vi "Is Error.vi"(8 "error in":errorcluster, 11 "Queue in":refnum<queue>) -> (0 "error out":errorcluster, 3 "Queue out":refnum<queue>)   [LabVIEW 2018, in "Module A.lvlib"]
doc: "Sends state machine to error case."
uses:
  Module A.lvlib
  ctl/Message Data--cluster.ctl
  ctl/State--enum.ctl
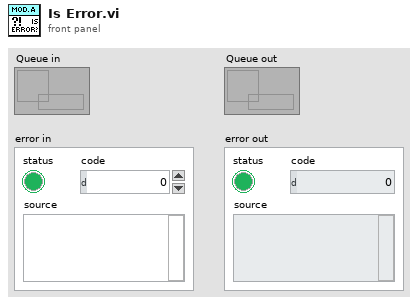
[diagram p1: front panel]
types:
  T1 = typedef "Module A.lvlib/State--enum.ctl" = enum16{"Initialize", "Error", "Shut Down", "Stop Module", "---", "Template", "Shut Module B", "Start Module B"}
  T2 = typedef "Module A.lvlib/Message Data--cluster.ctl" = cluster{"State":T1, "Data":variant}
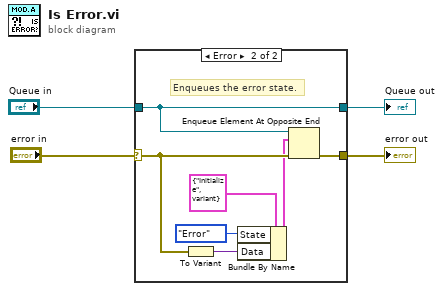
[diagram p0: block diagram]
diagram:
  n1 = case shown="Error" "error in" {
    selector: "error in" -> [w6 w9]
    tunnel: [w6 w8] -> w2
    tunnel: [w5 w13] -> w3
    tunnel: "Queue in" -> [w5 w13]
    frame No Error {
    }
    frame Error {
      # "Enqueues the error state."
      n2 = To Variant(anything=w9) -> (Variant=w10:variant)
      n3 = Bundle By Name(cluster=T2 {"State"=enum."Initialize", "Data"=variant} ("Message Data--cluster"), "State"=State--enum."Error", "Data"=w10) -> (w7:T2)
      n4 = Enqueue Element At Opposite End(queue=w13, element=w7, error in (no error)=w9) -> (error out=w8:errorcluster)  [unwired: 1 in, 2 out]
    }
  }
  "Queue out" <- w3
  "error out" <- w2
